vi "gm_measuringpoint_enable.vi"(8 "shift reg":u32, 9 "measuring point":u32, 10 "measuring mode":u8) -> (1 "shift reg out":u32, 2 "measuring point":u32)   [LabVIEW 2011]
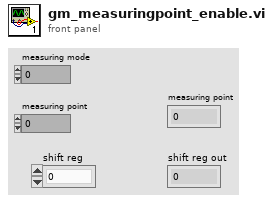
[diagram p1: front panel]
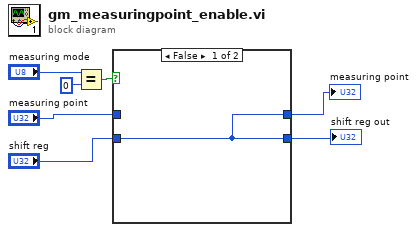
[diagram p0: block diagram]
diagram:
  n1 = Equal?(x="measuring mode", y=u8 0) -> (x = y?=w4:bool)
  n2 = case shown="False" w4 {
    tunnel: [w8 w9] -> w7
    tunnel: "measuring point" -> [_ w9]
    tunnel: "shift reg" -> [w8 _]
    tunnel: [w8 w9] -> w1
    frame False {
    }
    frame True {
    }
  }
  "shift reg out" <- w7
  "measuring point" <- w1
